vi "HK Channel Save Settings.vi"(8 "error in (no error)":errorcluster, 11 "HK Channel in":refnum<class "HK Table.lvclass">) -> (0 "error out":errorcluster, 2 "Channel List":T1[](array[typedef]), 3 "HK Channel out":refnum<class "HK Table.lvclass">)   [LabVIEW 2024, in "HK Table.lvclass"]
uses:
  HK Table.lvclass
  HK Channel Settings.ctl
  HK Item/HK Channel Units and Setup.ctl
  HK Item/HK Channel enum Data Type.ctl
  HK Item/HK Channel Settings Scaling.ctl
  HK Item/HK Channel enum Scaling Type.ctl
  HK Item/HK Channel Settings Physical.ctl
  HK Item/HK Channel Settings Limits.ctl
  HK Alarms/HK Channel Settings Alarms.ctl
  HK Alarms/HK Alarm enum Action.ctl
  HK Table.lvclass/HK Table.ctl
  HK Item/HK Item.lvclass/HK Item.ctl
  HK Alarms/HK Alarms.lvclass/HK Alarms.ctl
  HK Alarms/HK Alarms.lvclass
  HK Item/HK Item.lvclass
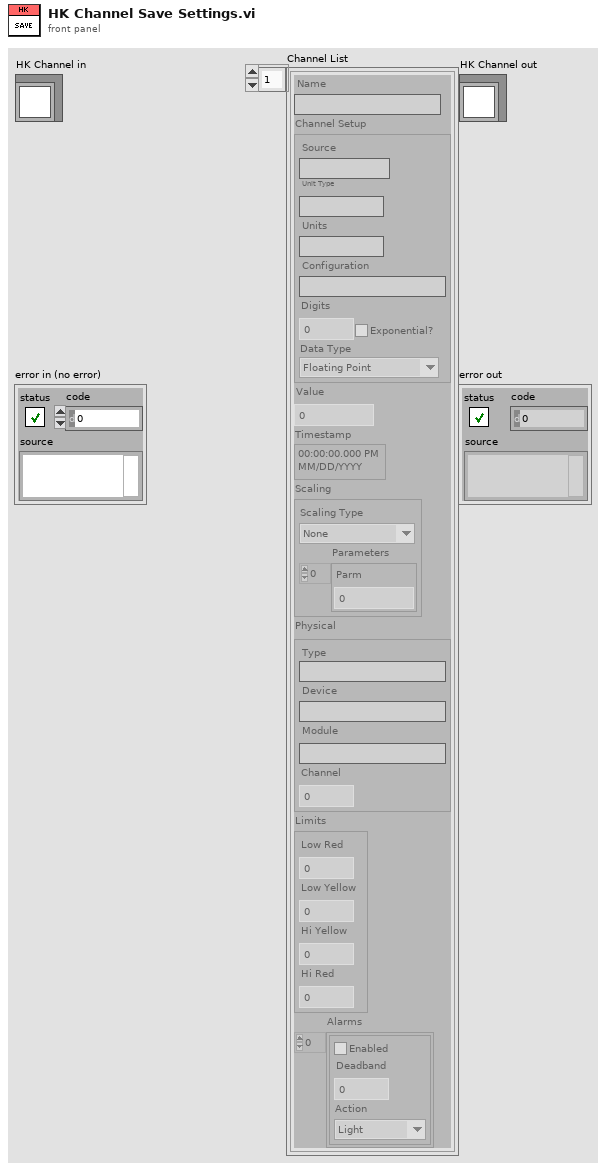
[diagram p1: front panel]
types:
  T1 = typedef "HK Table.lvclass/HK Channel Settings.ctl" = cluster{"Name":string, "Channel Setup":T2, "Value":dbl, "Timestamp":timestamp, "Scaling":T4, "Physical":T6, "Limits":T7, "Alarms":T8[]}
  T2 = typedef "HK Item.lvclass/HK Channel Units and Setup.ctl" = cluster{"Unit Type":string, "Units":string, "Configuration":string, "Digits":i32, "Data Type":T3, "Exponential?":bool, "Source":string}
  T3 = typedef "HK Item.lvclass/HK Channel enum Data Type.ctl" = enum16{"Floating Point", "Integer", "Enum", "String", "Waveform", "File"}
  T4 = typedef "HK Item.lvclass/HK Channel Settings Scaling.ctl" = cluster{"Scaling Type":T5, "Parameters":dbl[]}
  T5 = typedef "HK Item.lvclass/HK Channel enum Scaling Type.ctl" = enum16{"None", "Polynomial"}
  T6 = typedef "HK Item.lvclass/HK Channel Settings Physical.ctl" = cluster{"Type":string, "Device":string, "Module":string, "Channel":i32}
  T7 = typedef "HK Item.lvclass/HK Channel Settings Limits.ctl" = cluster{"Low Red":dbl, "Low Yellow":dbl, "Hi Yellow":dbl, "Hi Red":dbl}
  T8 = typedef "HK Item.lvclass/HK Channel Settings Alarms.ctl" = cluster{"Enabled":bool, "Deadband":i32, "Action":T9}
  T9 = typedef "HK Item.lvclass/HK Alarm enum Action.ctl" = enum16{"Light", "Message", "Safe"}
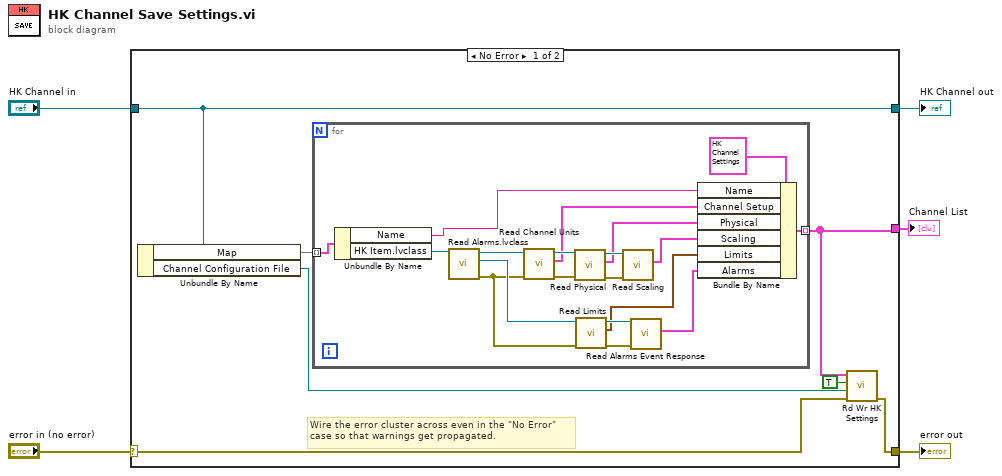
[diagram p0: block diagram]
diagram:
  n1 = case shown="No Error" "error in (no error)" {
    selector: "error in (no error)" -> [w10 w33]
    tunnel: [w9 w33] -> w4
    tunnel: [w12 w32] -> w2
    tunnel: "HK Channel in" -> [w12 w32]
    tunnel: [w8 _] -> w1
    frame No Error {
      # "Wire the error cluster across even in the \"No Error\"\ncase so that warnings get propagated."
      n2 = Unbundle By Name(w12) -> ("Map"=w11:map{string, refnum<class "HK Item.lvclass">}, "Channel Configuration File"=w7:path)
      n3 = for {
        tunnel: w11 -> [w31] mode=indexing
        tunnel: [w13] -> w8 mode=indexing
        n4 = Unbundle By Name(w31) -> ("Name"=w24:string, "HK Item.lvclass"=w28:refnum<class "HK Item.lvclass">)
        n5 = call "Read Alarms.lvclass.vi"("HK Item in"=w28) -> ("error out"=w17:errorcluster, "Alarms.lvclass"=w22:refnum<class "HK Alarms.lvclass">, "HK Item out"=w27:refnum<class "HK Item.lvclass">)  [unwired: 8 in]
        n6 = call "Read Channel Units.vi"("error in (no error)"=w17, "HK Item in"=w27) -> ("error out"=w19:errorcluster, "Channel Setup"=w23:T2, "HK Item out"=w30:refnum<class "HK Item.lvclass">)  [unwired: 7 in]
        n7 = call "Read Physical.vi"("error in (no error)"=w19, "HK Item in"=w30) -> ("error out"=w18:errorcluster, "Physical"=w21:T6, "HK Item out"=w29:refnum<class "HK Item.lvclass">)  [unwired: 7 in]
        n8 = call "Read Limits.vi"("error in (no error)"=w17, "Alarms in"=w22) -> ("error out"=w16:errorcluster, "Limits"=w14:T7, "Alarms out"=w26:refnum<class "HK Alarms.lvclass">)  [unwired: 7 in]
        n9 = call "Read Scaling.vi"("error in (no error)"=w18, "HK Item in"=w29) -> ("Scaling"=w20:T4)  [unwired: 7 in, 2 out]
        n10 = call "Read Alarms Event Response.vi"("error in (no error)"=w16, "Alarms in"=w26) -> ("Alarms"=w15:T8[])  [unwired: 7 in, 2 out]
        n11 = Bundle By Name(cluster=T1 {"Name"="", "Channel Setup"={"Unit Type"="", "Units"="", "Configuration"="", "Digits"=0, "Data Type"=enum."Floating Point", "Exponential?"=FALSE, "Source"=""}, "Value"=0.0, "Timestamp"=timestamp(0 s since 1904-01-01), "Scaling"={"Scaling Type"=enum."None", "Parameters"=[]}, "Physical"={"Type"="", "Device"="", "Module"="", "Channel"=0}, "Limits"={"Low Red"=0.0, "Low Yellow"=0.0, "Hi Yellow"=0.0, "Hi Red"=0.0}, "Alarms"=[]} ("channel settings"), "Name"=w24, "Channel Setup"=w23, "Physical"=w21, "Scaling"=w20, "Limits"=w14, "Alarms"=w15) -> (w13:T1)
      }
      n12 = call "Rd Wr HK Settings.vi"("error in (no error)"=w10, "File Path"=w7, "Write? (F:Read)"=TRUE, "channels"=w8) -> ("error out"=w9:errorcluster)  [unwired: 6 in, 1 out]
    }
    frame Error {
    }
  }
  "error out" <- w4
  "HK Channel out" <- w2
  "Channel List" <- w1
